vi "Global Oscillator Frequency.vi"() -> ()   [LabVIEW 2019]
panel:
  in  "Oscillator Frequency Global":dbl=3686400.0
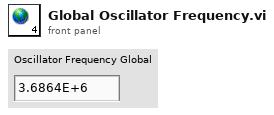
[diagram p1: front panel]
diagram:
